vi "EX4 correction.vi"() -> ()   [LabVIEW 2018]
panel:
  in  "Numeric":i8 min=0 max=6
  out "Boolean 7":bool
  out "Boolean 6":bool
  out "Boolean 5":bool
  out "Boolean 4":bool
  out "Boolean 3":bool
  out "Boolean 2":bool
  out "Boolean":bool
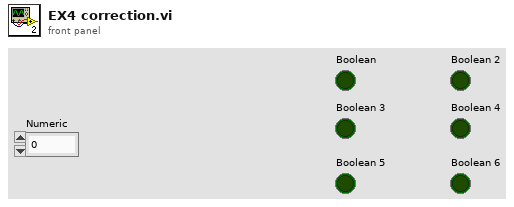
[diagram p1: front panel]
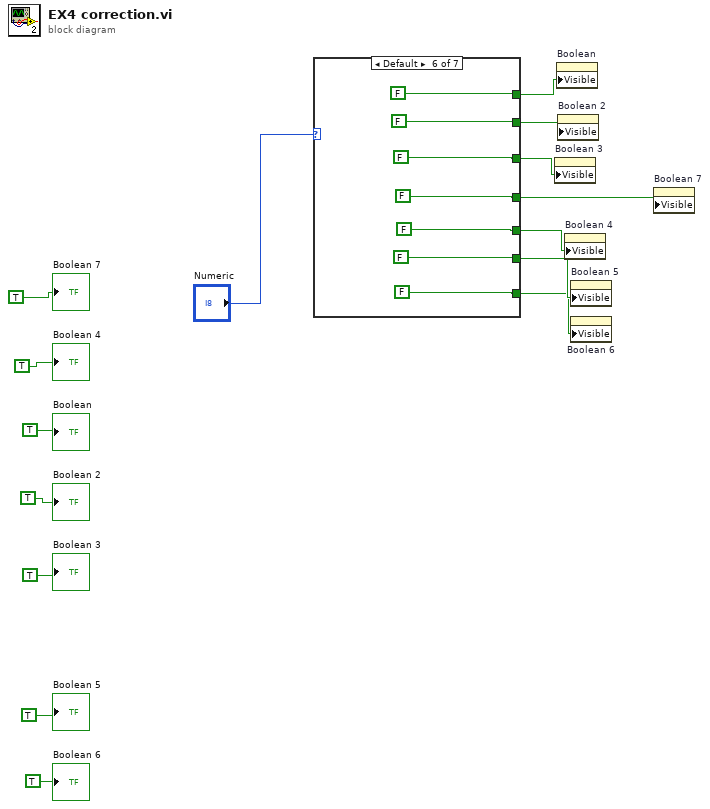
[diagram p0: block diagram]
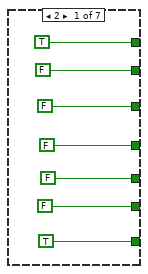
[diagram p2: hidden frame]
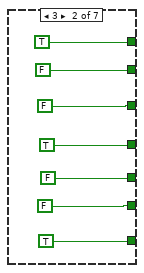
[diagram p3: hidden frame]
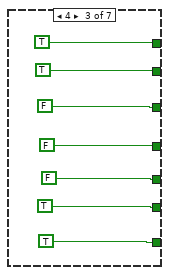
[diagram p4: hidden frame]
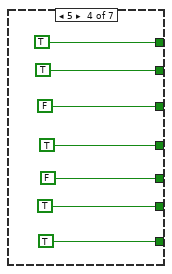
[diagram p5: hidden frame]
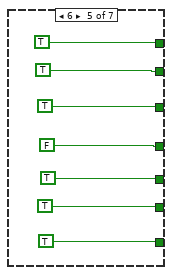
[diagram p6: hidden frame]
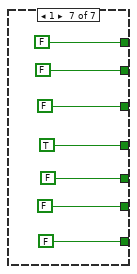
[diagram p7: hidden frame]
diagram:
  n1 = case shown="Default" "Numeric" {
    tunnel: [FALSE FALSE TRUE TRUE TRUE FALSE FALSE] -> w13
    tunnel: [FALSE FALSE FALSE FALSE TRUE FALSE FALSE] -> w12
    tunnel: [FALSE TRUE FALSE TRUE FALSE FALSE TRUE] -> w11
    tunnel: [FALSE FALSE FALSE FALSE TRUE FALSE FALSE] -> w10
    tunnel: [FALSE FALSE TRUE TRUE TRUE FALSE FALSE] -> w9
    tunnel: [TRUE TRUE TRUE TRUE TRUE FALSE FALSE] -> w8
    tunnel: [TRUE TRUE TRUE TRUE TRUE FALSE FALSE] -> w14
    frame 2 {
    }
    frame 3 {
    }
    frame 4 {
    }
    frame 5 {
    }
    frame 6 {
    }
    frame Default {
    }
    frame 1 {
    }
  }
  n2 = property on="Boolean 3" class="Bool (strict)"("Visible"=w12) -> ()  [unwired: 2 in, 2 out]
  n3 = property on="Boolean" class="Bool (strict)"("Visible"=w14) -> ()  [unwired: 2 in, 2 out]
  n4 = property on="Boolean 2" class="Bool (strict)"("Visible"=w13) -> ()  [unwired: 2 in, 2 out]
  n5 = property on="Boolean 4" class="Bool (strict)"("Visible"=w10) -> ()  [unwired: 2 in, 2 out]
  n6 = property on="Boolean 5" class="Bool (strict)"("Visible"=w9) -> ()  [unwired: 2 in, 2 out]
  n7 = property on="Boolean 6" class="Bool (strict)"("Visible"=w8) -> ()  [unwired: 2 in, 2 out]
  n8 = property on="Boolean 7" class="Bool (strict)"("Visible"=w11) -> ()  [unwired: 2 in, 2 out]
  "Boolean" <- TRUE
  "Boolean 2" <- TRUE
  "Boolean 3" <- TRUE
  "Boolean 4" <- TRUE
  "Boolean 5" <- TRUE
  "Boolean 6" <- TRUE
  "Boolean 7" <- TRUE
